vi "poziomy.vi"(6 "error in (no error)":errorcluster, 8 "Akcja":T7=enum."Reset ramienia", 9 "LINX Resource in":T1) -> (0 "error out":errorcluster, 1 "KONIEC":bool, 2 "Aktualny stan":T8, 3 "LINX Resource out":T1)   [LabVIEW 2014]
uses:
  poziomyVIs/RuchPoziomy.ctl
  wczytajDaneDoRuchuVIs/Akcje_wczytywania_danych_do_ruchu.ctl
  <vilib>/MakerHub/LINX/Private/Type Defs/LINX Ref.ctl
  <vilib>/MakerHub/LINX/Private/Type Defs/Platform.ctl
  <vilib>/MakerHub/LINX/Private/Type Defs/Interface.ctl
  <vilib>/MakerHub/LINX/Private/Device/Type Defs/LINX Device Config.ctl
  <vilib>/MakerHub/LINX/Private/Device/Type Defs/TCP Config.ctl
  <vilib>/MakerHub/LINX/Private/Device/Type Defs/Channels.ctl
  poziomyVIs/WspolrzednaPoz.ctl
  Akcja_kontrolki.ctl
  Faza_ruchu.ctl
  gotowoscDoPomiaruVIs/wczytaj_zapisz.ctl
  <vilib>/MakerHub/LINX/Public/Peripherals/Digital/Digital Read 1 Chan.vi
  <vilib>/MakerHub/LINX/Public/Peripherals/Digital/Digital Read N Chans.vi
  <vilib>/MakerHub/LINX/Private/Local IO/LinxDigitalRead.vi
  <vilib>/MakerHub/LINX/Public/Utilities/Check Channel.vi
  <vilib>/MakerHub/LINX/Private/Local IO/Handle Errors.vi
  <vilib>/MakerHub/LINX/Private/Utilties/Generate Error.vi
  <vilib>/MakerHub/LINX/LMH-LINX.lvlib
  <vilib>/MakerHub/LINX/Private/Device/Device.lvlib
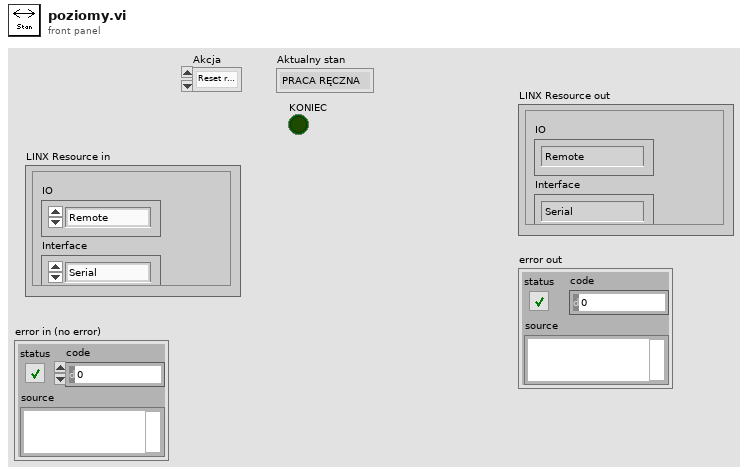
[diagram p1: front panel]
types:
  T1 = typedef "LMH-LINX.lvlib/LINX Ref.ctl" = cluster{"IO":T2, "Interface":T3, "LINX Device Config":T4}
  T2 = typedef "LMH-LINX.lvlib/Platform.ctl" = enum16{"Remote", "Local"}
  T3 = typedef "LMH-LINX.lvlib/Interface.ctl" = enum16{"Serial", "TCP"}
  T4 = typedef "LMH-LINX.lvlib/Device.lvlib/LINX Device Config.ctl" = cluster{"Interface":T3, "COM Port":refnum<visa-resource-name>, "TCP Configuration":T5, "Device Family":u8, "Device ID":u8, "Device Name":string, "TCP Ref":refnum<k5>, "Channels":T6}
  T5 = typedef "LMH-LINX.lvlib/Device.lvlib/TCP Config.ctl" = cluster{"IP Address":string, "Port":u16}
  T6 = typedef "LMH-LINX.lvlib/Channels.ctl" = cluster{"DI":u8[], "DO":u8[], "AI":u8[], "AO":u8[], "PWM":u8[], "QE":u8[], "UART":u8[], "I2C 2":u8[], "SPI":u8[], "CAN":u8[], "Servo":u8[], "AI Ref (V)":dbl, "AI Resolution (Bits)":u8, "AO Ref (V)":dbl, "AO Resolution (Bits)":u8}
  T7 = typedef "Akcje_wczytywania_danych_do_ruchu.ctl" = enum16{"Init", "Reset ramienia", "Przygotuj listę", "Sprawdź"}
  T8 = typedef "RuchPoziomy.ctl" = enum16{"PRACA RĘCZNA", "COFAJ", "NAPRZÓD", "WYŁ."}
  T9 = typedef "WspolrzednaPoz.ctl" = cluster{"Stan poziomy":T8, "Pozycja":i32}
  T10 = typedef "Akcja_kontrolki.ctl" = enum16{"Czytaj", "Zapisz", "Reset"}
  T11 = typedef "wczytaj_zapisz.ctl" = enum16{"Zapisz", "Wczytaj"}
  T12 = typedef "Faza_ruchu.ctl" = enum16{"Ruch", "Poczekaj", "Pomiar"}
  T13 = typedef "Diody_zbior.ctl" = cluster{"Lewo":bool, "Prawo":bool, "Góra":bool, "Dół":bool, "Działanie":bool, "Czujnik":bool, "Pomiar":bool}
  T14 = typedef "Przyciski_zbior.ctl" = cluster{"LEWO":bool, "PRAWO":bool, "GÓRA":bool, "Dӣ":bool, "Stop":bool, "Start":bool, "Praca ręczna":bool}
  T15 = typedef "Gotowosc.ctl" = cluster{"Poziomy":bool, "Pionowy":bool}
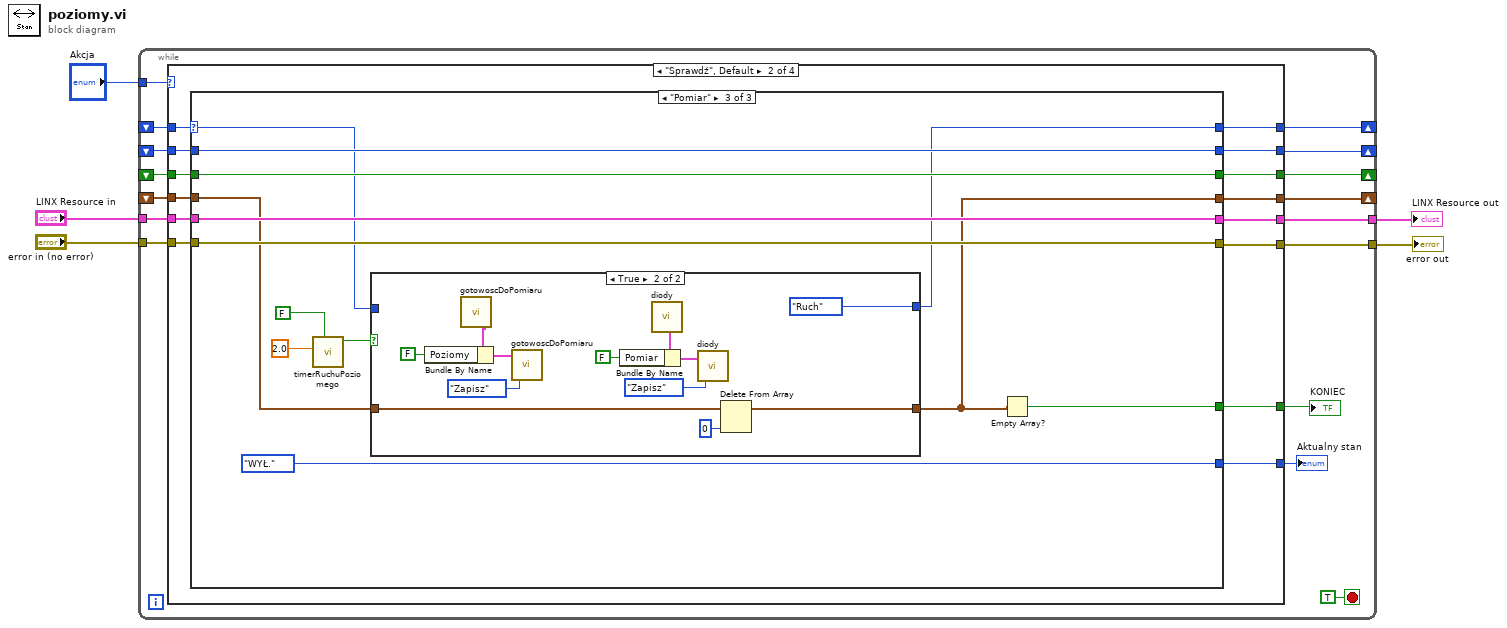
[diagram p0: block diagram]
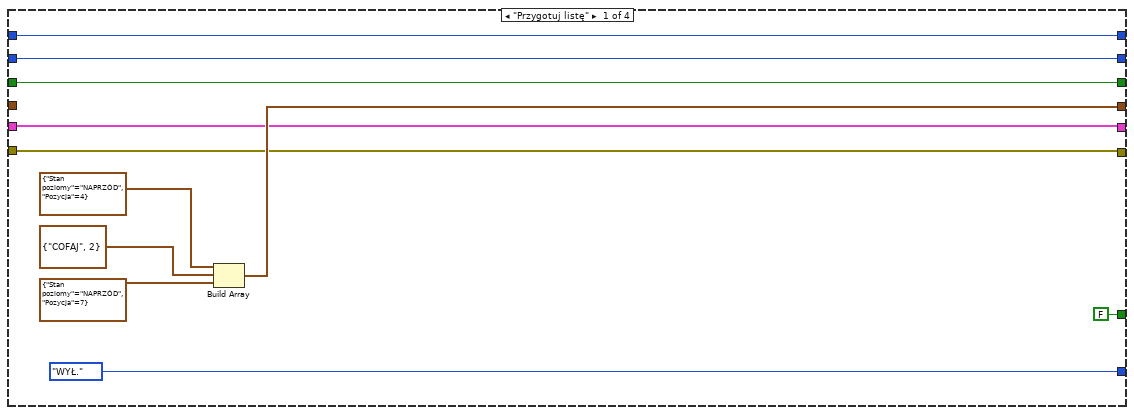
[diagram p2: hidden frame]
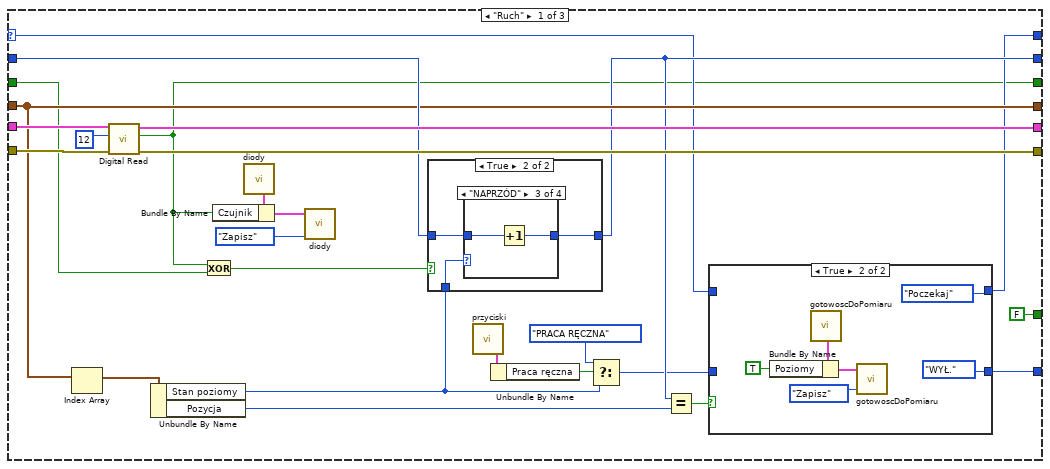
[diagram p3: hidden frame]
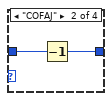
[diagram p7: hidden frame]
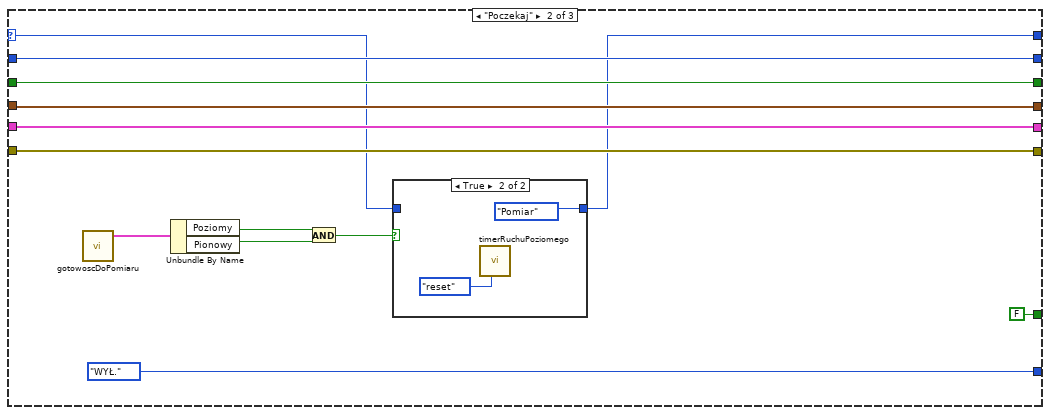
[diagram p9: hidden frame]
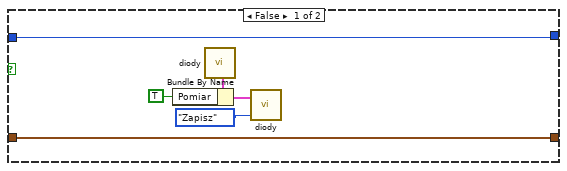
[diagram p11: hidden frame]
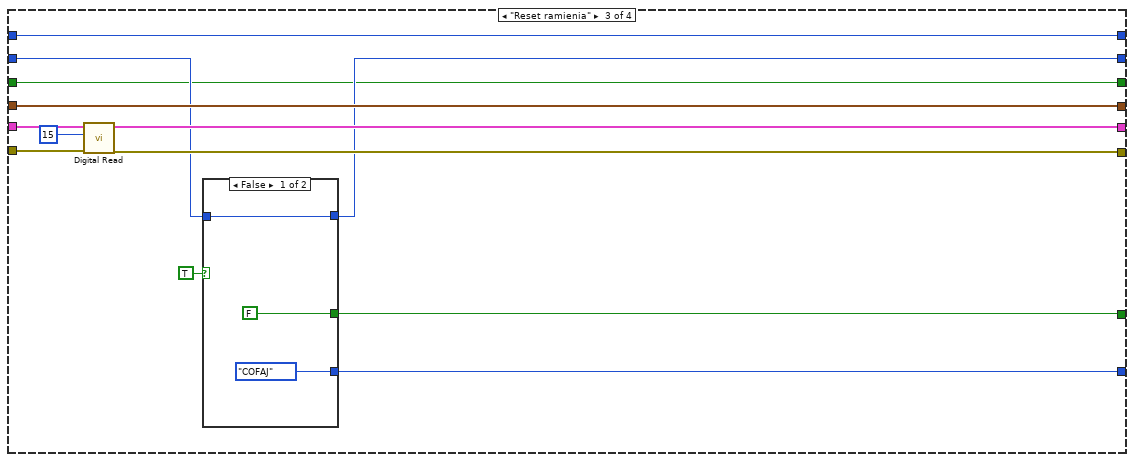
[diagram p12: hidden frame]
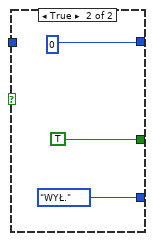
[diagram p13: hidden frame]
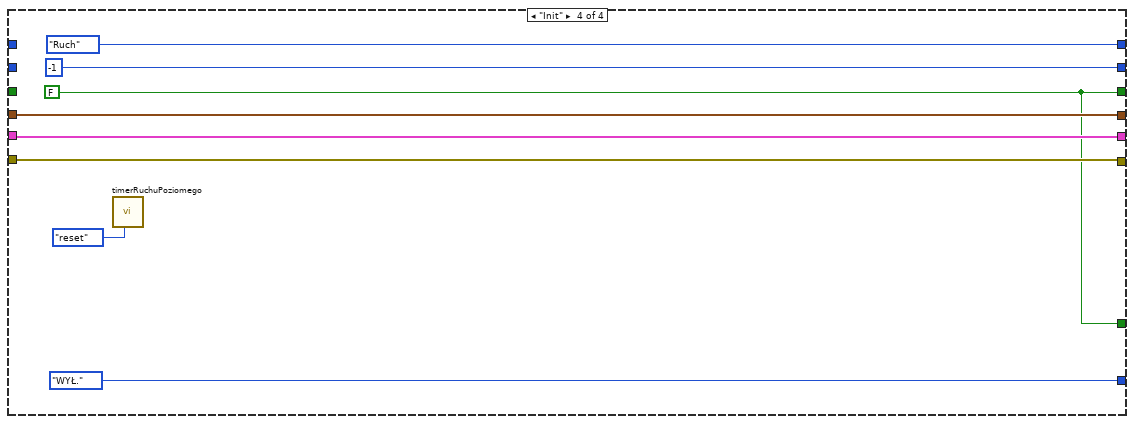
[diagram p14: hidden frame]
diagram:
  n1 = while {
    shift-right: [w19] -> _
    shift-left: _ -> [w20]
    tunnel: "Akcja" -> [w18]
    tunnel: "LINX Resource in" -> [w17]
    tunnel: [w15] -> w3
    tunnel: "error in (no error)" -> [w16]
    tunnel: [w14] -> w1
    shift-right: [w13] -> _
    shift-left: _ -> [w11]
    shift-right: [w12] -> _
    shift-left: _ -> [w10]
    shift-right: [w9] -> _
    shift-left: _ -> [w8]
    stop <- TRUE stop-if-true
    n2 = case shown="\"Sprawdź\", Default" w18 {
      tunnel: w20 -> [_ w38 w150 w161]
      tunnel: [w32 w36 w150 w161] -> w19
      tunnel: w17 -> [w31 w46 w148 w160]
      tunnel: w16 -> [w30 w44 w146 w159]
      tunnel: [w31 w45 w147 w160] -> w15
      tunnel: [w30 w43 w145 w159] -> w14
      tunnel: [w23 w41 w140 w157] -> w13
      tunnel: [w29 w39 w143 -1] -> w12
      tunnel: w11 -> [w23 w42 w140 _]
      tunnel: w10 -> [w29 w40 w141 _]
      tunnel: [w24 w35 w149 Faza_ruchu."Ruch" ("Faza ruchu")] -> w9
      tunnel: w8 -> [w24 w37 w149 _]
      tunnel: [RuchPoziomy."WYŁ." ("Stan poziomy") w34 w142 RuchPoziomy."WYŁ." ("Stan poziomy")] -> w7
      tunnel: [FALSE ("empty?") w33 w138 w157] -> w6
      frame "Przygotuj listę" {
        n3 = Build Array(T9 {"Stan poziomy"=enum."NAPRZÓD", "Pozycja"=4} ("Cluster"), T9 {"Stan poziomy"=enum."COFAJ", "Pozycja"=2} ("Cluster"), T9 {"Stan poziomy"=enum."NAPRZÓD", "Pozycja"=7} ("Cluster")) -> (w32:T9[])
      }
      frame "Sprawdź", Default {
        n4 = case shown="\"Pomiar\"" w37 {
          selector: w37 -> [w53 w93 w112]
          tunnel: w46 -> [w72 w100 w116]
          tunnel: [w71 w100 w116] -> w45
          tunnel: w44 -> [w66 w99 w115]
          tunnel: [w65 w99 w115] -> w43
          tunnel: w42 -> [w50 w102 w117]
          tunnel: [w49 w102 w117] -> w41
          tunnel: w40 -> [w63 w103 w118]
          tunnel: [w54 w103 w118] -> w39
          tunnel: w38 -> [w62 w101 w110]
          tunnel: [w62 w101 w108] -> w36
          tunnel: [w52 w92 w111] -> w35
          tunnel: [w48 RuchPoziomy."WYŁ." ("Stan poziomy") RuchPoziomy."WYŁ." ("Stan poziomy")] -> w34
          tunnel: [FALSE ("empty?") FALSE ("empty?") w107] -> w33
          frame "Ruch" {
            n5 = Index Array(array=w62) -> (element=w61:T9)  [unwired: 1 in]
            n6 = call-poly <vilib>:"Digital Read.vi"("Error In"=w66, "DI Channel"=u8 12, "LINX Resource"=w72) -> ("Error Out"=w65:errorcluster, "DI Value"=w49:bool, "LINX Resource"=w71:T1)  [unwired: 6 in]
            n7 = Unbundle By Name(w61) -> ("Stan poziomy"=w59:T8, "Pozycja"=w60:i32)
            n8 = Exclusive Or(1:w50, 2:w49) -> (0:w64:bool)
            n9 = call "diody.vi"() -> ("Wyjście"=w68:T13)  [unwired: 5 in]
            n10 = Bundle By Name(cluster=w68, "Czujnik"=w49) -> (w67:T13)
            n11 = call "diody.vi"("Akcja"=Akcja_kontrolki."Zapisz", "Wejście"=w67) -> ()  [unwired: 3 in, 1 out]
            n12 = case shown="True" w64 {
              tunnel: w63 -> [w81 w84]
              tunnel: [w81 w83] -> w54
              tunnel: w59 -> [_ w82]
              frame False {
              }
              frame True {
                n13 = case shown="\"NAPRZÓD\"" w82 {
                  tunnel: w84 -> [w85 w87 w89 w90]
                  tunnel: [w85 w86 w88 w90] -> w83
                  frame "PRACA RĘCZNA" {
                  }
                  frame "COFAJ" {
                    n14 = Decrement(x=w87) -> (x-1=w86:i32)
                  }
                  frame "NAPRZÓD" {
                    n15 = Increment(x=w89) -> (x+1=w88:i32)
                  }
                  frame "WYŁ." {
                  }
                }
              }
            }
            n16 = call "przyciski.vi"() -> ("Wyjście"=w56:T14)  [unwired: 5 in]
            n17 = Unbundle By Name(w56) -> ("Praca ręczna"=w58:bool)
            n18 = Select(t=RuchPoziomy."PRACA RĘCZNA" ("Stan pracy ręcznej - poz"), s=w58, f=w59) -> (s? t:f=w51:T8)
            n19 = Equal?(x=w54, y=w60) -> (x = y?=w55:bool)
            n20 = case shown="True" w55 {
              tunnel: w53 -> [w74 _]
              tunnel: [w74 Faza_ruchu."Poczekaj" ("f")] -> w52
              tunnel: w51 -> [w73 _]
              tunnel: [w73 RuchPoziomy."WYŁ." ("Stan poziomy")] -> w48
              frame False {
              }
              frame True {
                n21 = call "gotowoscDoPomiaru.vi"() -> ("Gotowość wyjście"=w78:T15)  [unwired: 5 in]
                n22 = Bundle By Name(cluster=w78, "Poziomy"=TRUE) -> (w79:T15)
                n23 = call "gotowoscDoPomiaru.vi"("Wczytaj_zapisz"=wczytaj_zapisz."Zapisz", "Gotowość"=w79) -> ()  [unwired: 3 in, 1 out]
              }
            }
          }
          frame "Poczekaj" {
            n24 = call "gotowoscDoPomiaru.vi"() -> ("Gotowość wyjście"=w96:T15)  [unwired: 5 in]
            n25 = Unbundle By Name(w96) -> ("Poziomy"=w98:bool, "Pionowy"=w97:bool)
            n26 = And(x=w98, y=w97) -> (x .and. y?=w94:bool)
            n27 = case shown="True" w94 {
              tunnel: w93 -> [w104 _]
              tunnel: [w104 Faza_ruchu."Pomiar" ("t")] -> w92
              frame False {
              }
              frame True {
                n28 = call "timerRuchuPoziomego.vi"("Czynność"=enum16{"reset", "działaj"}."reset") -> ()  [unwired: 10 in, 1 out]
              }
            }
          }
          frame "Pomiar" {
            n29 = call "timerRuchuPoziomego.vi"("pauza"=FALSE, "Czas"=2.0) -> ("czy czas upłynął"=w113:bool)  [unwired: 9 in]
            n30 = case shown="True" w113 {
              tunnel: w112 -> [w125 _]
              tunnel: [w125 Faza_ruchu."Ruch" ("Faza ruchu")] -> w111
              tunnel: w110 -> [w124 w132]
              tunnel: [w124 w131] -> w108
              frame False {
                n31 = call "diody.vi"() -> ("Wyjście"=w123:T13)  [unwired: 5 in]
                n32 = Bundle By Name(cluster=w123, "Pomiar"=TRUE) -> (w121:T13)
                n33 = call "diody.vi"("Akcja"=Akcja_kontrolki."Zapisz", "Wejście"=w121) -> ()  [unwired: 3 in, 1 out]
              }
              frame True {
                n34 = call "gotowoscDoPomiaru.vi"() -> ("Gotowość wyjście"=w135:T15)  [unwired: 5 in]
                n35 = Bundle By Name(cluster=w135, "Poziomy"=FALSE) -> (w136:T15)
                n36 = call "gotowoscDoPomiaru.vi"("Wczytaj_zapisz"=wczytaj_zapisz."Zapisz", "Gotowość"=w136) -> ()  [unwired: 3 in, 1 out]
                n37 = call "diody.vi"() -> ("Wyjście"=w129:T13)  [unwired: 5 in]
                n38 = Bundle By Name(cluster=w129, "Pomiar"=FALSE) -> (w127:T13)
                n39 = call "diody.vi"("Akcja"=Akcja_kontrolki."Zapisz", "Wejście"=w127) -> ()  [unwired: 3 in, 1 out]
                n40 = Delete From Array(array=w132, index=0) -> (array with subset deleted=w131:T9[])  [unwired: 1 in, 1 out]
              }
            }
            n41 = Empty Array?(array=w108) -> (empty?=w107:bool)
          }
        }
      }
      frame "Reset ramienia" {
        n42 = call-poly <vilib>:"Digital Read.vi"("Error In"=w146, "DI Channel"=u8 15, "LINX Resource"=w148) -> ("Error Out"=w145:errorcluster, "LINX Resource"=w147:T1)  [unwired: 6 in, 1 out]
        n43 = case shown="False" TRUE {
          tunnel: [w152 0] -> w143
          tunnel: [RuchPoziomy."COFAJ" ("Stan poziomy") RuchPoziomy."WYŁ." ("Stan poziomy")] -> w142
          tunnel: w141 -> [w152 _]
          tunnel: [FALSE TRUE] -> w138
          frame False {
          }
          frame True {
          }
        }
      }
      frame "Init" {
        w157 = FALSE
        n44 = call "timerRuchuPoziomego.vi"("Czynność"=enum16{"reset", "działaj"}."reset") -> ()  [unwired: 10 in, 1 out]
      }
    }
    "Aktualny stan" <- w7
    "KONIEC" <- w6
  }
  "error out" <- w1
  "LINX Resource out" <- w3
